vi "Configure Session.vi"(8 "error in":errorcluster, 11 "Plugin in":refnum<class "AutomotiveDataSimulator.lvclass">) -> (0 "error out":errorcluster, 3 "Plugin out":refnum<class "AutomotiveDataSimulator.lvclass">)   [LabVIEW 2020, in "AutomotiveDataSimulator.lvlib" / "AutomotiveDataSimulator.lvclass"]
uses:
  AutomotiveDataSimulator.lvclass
  C:/Program Files/National Instruments/LabVIEW 2020/vi.lib/FlexLogger/SDK/PluginSDK.lvlibp/PEFClasses/SDK/Plugin/Plugin.lvclass
  AutomotiveDataSimulator.lvclass/AutomotiveDataSimulator.ctl
  <vilib>/FlexLogger/SDK/PluginSDK.lvlibp/PEFClasses/SDK/Plugin/ParameterAccess/Read Enum.vi
  <vilib>/FlexLogger/SDK/PluginSDK.lvlibp/PEFClasses/SDK/Plugin/Plugin.lvclass
  C:/Program Files/National Instruments/LabVIEW 2020/vi.lib/FlexLogger/SDK/PluginSDK.lvlibp/PEFClasses/SDK/Processing Element/Processing Element.lvclass
  C:/Users/dgrajale/Desktop/Flexlogger Project/Flexlogger Plugins/AutomotiveDataSimulator/AutomotiveDataSimulator.lvclass
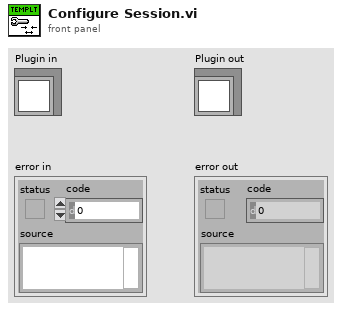
[diagram p1: front panel]
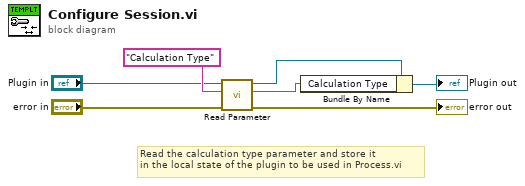
[diagram p0: block diagram]
diagram:
  # "Read the calculation type parameter and store it\nin the local state of the plugin to be used in Process.vi"
  n1 = call-poly <vilib>:"Read Parameter.vi"("error in (no error)"="error in", "Name"="Calculation Type", "Plugin in"="Plugin in") -> ("error out"=→"error out":errorcluster, "Value"=w2:string, "Plugin out"=w4:refnum<class "AutomotiveDataSimulator.lvclass">)  [unwired: 4 in, 2 out]
  n2 = Bundle By Name(cluster=w4, "Calculation Type"=w2) -> (→"Plugin out":refnum<class "AutomotiveDataSimulator.lvclass">)
